vi "DT_Merge_Add Triangle.vi"(6 "left/right pt (right:F)":bool, 8 "point":i32, 9 "triangle":i32, 10 "Data In":T1, 11 "Triangles In":i32[][](array[numeric])) -> (2 "Data Out":T1, 3 "Triangles Out":i32[][](array[numeric]))   [LabVIEW 2020, in "NI_AAL_Geometry.lvlib"]
uses:
  <vilib>/Analysis/NI_AAL_Geometry.lvlib
  <vilib>/Analysis/geometry.llb/DT_Merge_Find Next Triangulation_Data.ctl
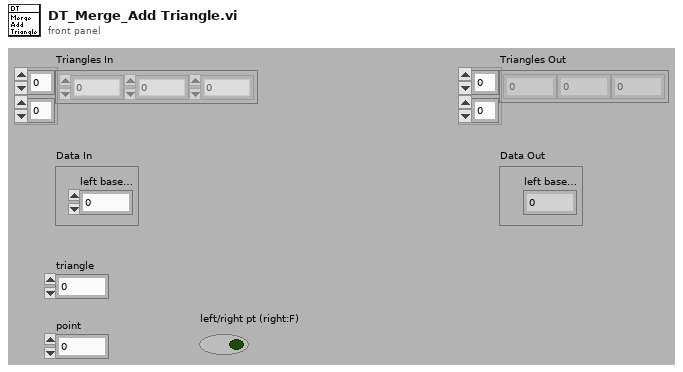
[diagram p1: front panel]
types:
  T1 = typedef "NI_AAL_Geometry.lvlib/DT_Merge_Find Next Triangulation_Data.ctl" = cluster{"left base point":i32, "left triangle":i32, "left local idx":i32, "right base point":i32, "right triangle":i32, "right local idx":i32, "Left Candidate Triangles":i32[], "Left Candidate Point Idx":i32[], "Right Candidate Triangles":i32[], "Right Candidate Point Idx":i32[], "cur triangle":i32}
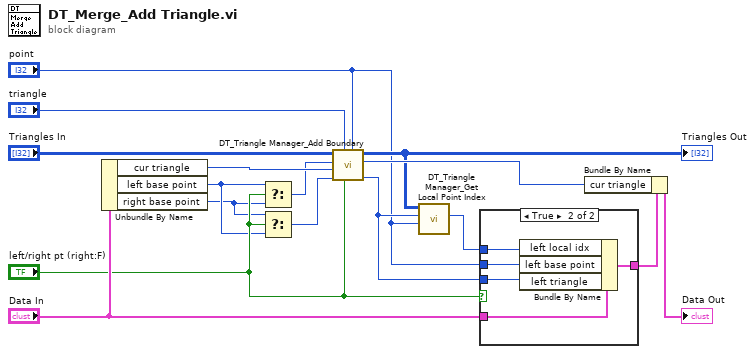
[diagram p0: block diagram]
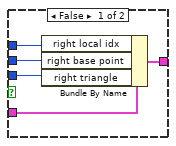
[diagram p2: hidden frame]
diagram:
  n1 = Unbundle By Name("Data In") -> ("cur triangle"=w16:i32, "left base point"=w6:i32, "right base point"=w1:i32)
  n2 = Select(t=w6, s="left/right pt (right:F)", f=w1) -> (s? t:f=w12:i32)
  n3 = Select(t=w1, s="left/right pt (right:F)", f=w6) -> (s? t:f=w11:i32)
  n4 = call <vilib>:"DT_Triangle Manager_Add Boundary.vi"("point 2"="point", "CCW? [T]"="left/right pt (right:F)", "triangle 2"="triangle", "point 1"=w11, "triangle 1"=w16, "apex point"=w12, "Triangles In"="Triangles In") -> ("new triangle 2"=w4:i32, "triangle"=w15:i32, "Triangles Out"=w5:i32[][])  [unwired: 2 out]
  "Triangles Out" <- w5
  n5 = call <vilib>:"DT_Triangle Manager_Get Local Point Index.vi"("global idx"="point", "triangle"=w4, "Triangles"=w5) -> ("local idx"=w2:i32)  [unwired: 8 out]
  n6 = case shown="True" "left/right pt (right:F)" {
    tunnel: "Data In" -> [w21 w26]
    tunnel: [w20 w25] -> w9
    tunnel: "point" -> [w19 w23]
    tunnel: w4 -> [w18 w24]
    tunnel: w2 -> [w17 w22]
    frame False {
      n7 = Bundle By Name(cluster=w21, "right local idx"=w17, "right base point"=w19, "right triangle"=w18) -> (w20:T1)
    }
    frame True {
      n8 = Bundle By Name(cluster=w26, "left local idx"=w22, "left base point"=w23, "left triangle"=w24) -> (w25:T1)
    }
  }
  n9 = Bundle By Name(cluster=w9, "cur triangle"=w15) -> (→"Data Out":T1)
